vi "ATM Controller.vi"(8 "error in (no error)":errorcluster) -> (0 "error out":errorcluster)   [LabVIEW 2012]
uses:
  TypeDefs/ATM Controller State.ctl
  TypeDefs/UI Items.ctl
  TypeDefs/User Console Commands.ctl
  TypeDefs/Error Classification.ctl
  TypeDefs/Simulated Database Command.ctl
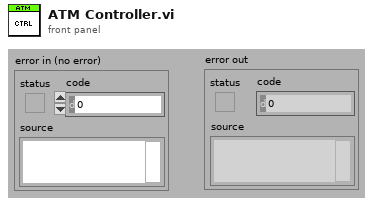
[diagram p1: front panel]
types:
  T1 = typedef "ATM Controller State.ctl" = enum16{"Initial", "Login", "Main Menu", "Balance Inquiry", "Deposit", "Deposit Complete", "Withdrawal", "Withdrawal Success", "Withdrawal Failure", "Terminate", "Lock Out"}
  T2 = typedef "User Console Commands.ctl" = enum16{"Init", "Set ATM Message", "Set ATM Menus", "Disable Controls", "Wait for Input", "Clear Keypad", "Return Card", "Close"}
  T3 = typedef "Error Classification.ctl" = enum16{"Minor", "Session", "System"}
  T4 = typedef "UI Items.ctl" = cluster{"Keypad":bool, "Card Slot":bool, "Left Buttons":bool, "Right Buttons":bool, "ATM Message":bool, "Left Menu":bool, "Right Menu":bool}
  T5 = typedef "Simulated Database Command.ctl" = enum16{"Init", "Look up and Lock Account", "Modify Balance", "Get Record", "Commit Record", "Unlock Record", "Close"}
  T6 = typedef "Record.ctl" = cluster{"Account Number":u32, "First Name":string, "Last Name":string, "Balance":dbl, "Locked":bool}
  T7 = typedef "UI to CTRL Command.ctl" = enum16{"Card Inserted", "Keypad Entry", "Button Pressed"}
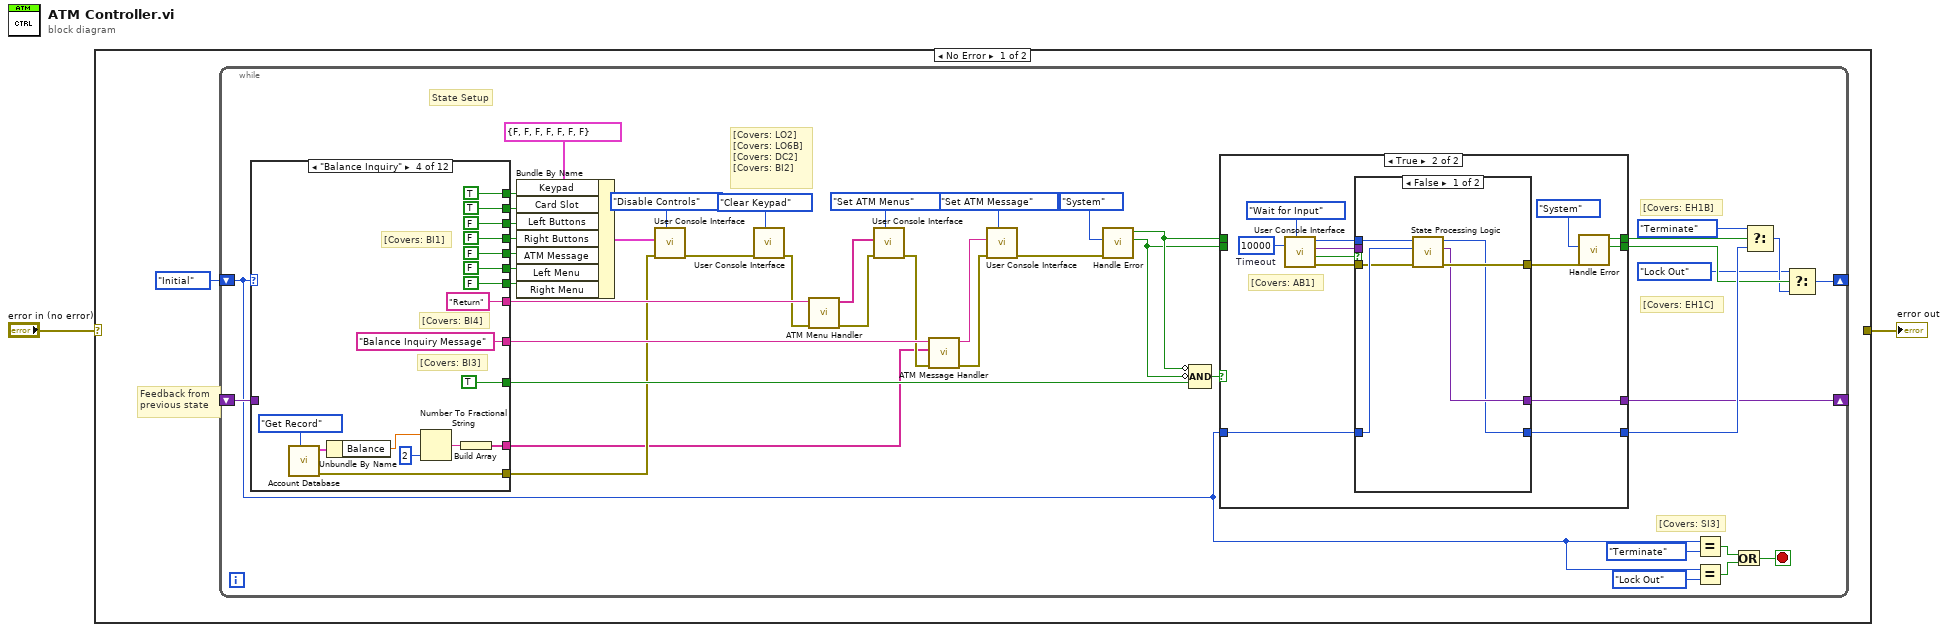
[diagram p0: block diagram]
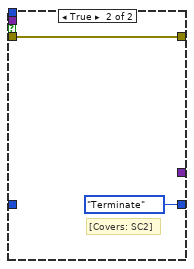
[diagram p3: hidden frame]
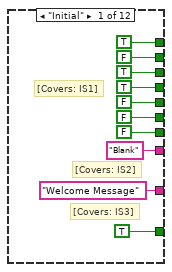
[diagram p4: hidden frame]
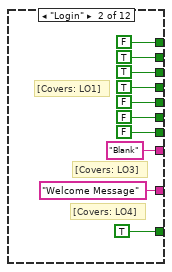
[diagram p5: hidden frame]
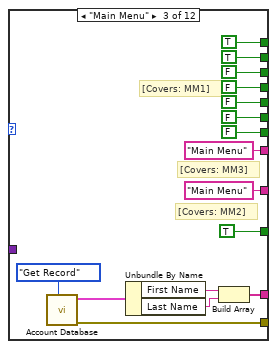
[diagram p6: hidden frame]
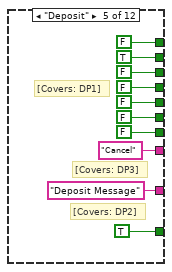
[diagram p7: hidden frame]
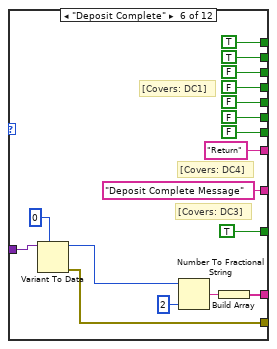
[diagram p8: hidden frame]
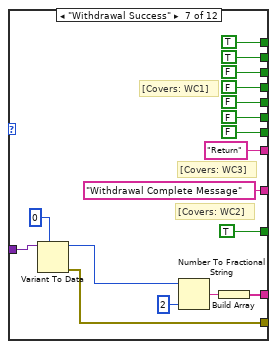
[diagram p9: hidden frame]
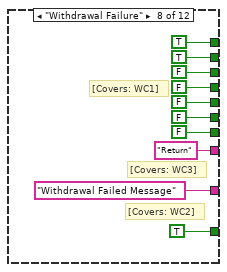
[diagram p10: hidden frame]
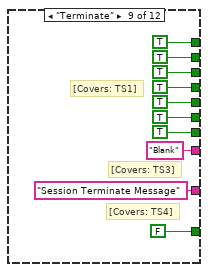
[diagram p11: hidden frame]
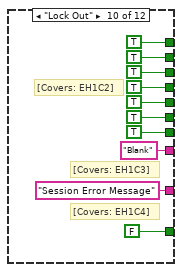
[diagram p12: hidden frame]
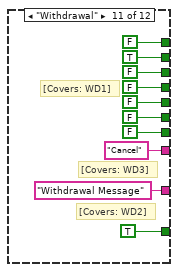
[diagram p13: hidden frame]
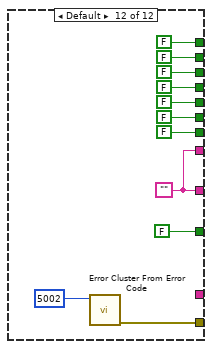
[diagram p14: hidden frame]
diagram:
  n1 = case shown="No Error" "error in (no error)" {
    selector: "error in (no error)" -> [_ w221]
    tunnel: [_ w221] -> w1
    frame No Error {
      # "Feedback from\nprevious state"
      n2 = while {
        shift-right: [w24] -> _
        shift-left: ATM_Controller_State."Initial" ("State") -> [w4]
        shift-right: [w11] -> _
        shift-left: _ -> [w10]
        stop <- w5 stop-if-true
        # "[Covers: SI3]"
        # "[Covers: LO2]\n[Covers: LO6B]\n[Covers: DC2]\n[Covers: BI2]"
        # "[Covers: EH1C]"
        # "[Covers: EH1B]"
        # "State Setup"
        n3 = case shown="\"Balance Inquiry\"" w4 {
          tunnel: [TRUE ("Keypad") FALSE ("Keypad") TRUE ("Keypad") TRUE ("Keypad") FALSE ("Keypad") TRUE ("Keypad") TRUE ("Keypad") TRUE ("Keypad") TRUE ("Keypad") TRUE ("Keypad") FALSE ("Keypad") FALSE ("Keypad")] -> w47
          tunnel: [FALSE ("Keypad") TRUE ("Keypad") TRUE ("Keypad") TRUE ("Keypad") TRUE ("Keypad") TRUE ("Keypad") TRUE ("Keypad") TRUE ("Keypad") TRUE ("Keypad") TRUE ("Keypad") TRUE ("Keypad") FALSE ("Keypad")] -> w46
          tunnel: [TRUE ("Keypad") TRUE ("Keypad") FALSE ("Keypad") FALSE ("Keypad") FALSE ("Keypad") FALSE ("Keypad") FALSE ("Keypad") FALSE ("Keypad") TRUE ("Keypad") TRUE ("Keypad") FALSE ("Keypad") FALSE ("Keypad")] -> w45
          tunnel: [TRUE ("Keypad") TRUE ("Keypad") FALSE ("Keypad") FALSE ("Keypad") FALSE ("Keypad") FALSE ("Keypad") FALSE ("Keypad") FALSE ("Keypad") TRUE ("Keypad") TRUE ("Keypad") FALSE ("Keypad") FALSE ("Keypad")] -> w44
          tunnel: [FALSE ("Keypad") FALSE ("Keypad") FALSE ("Keypad") FALSE ("Keypad") FALSE ("Keypad") FALSE ("Keypad") FALSE ("Keypad") FALSE ("Keypad") TRUE ("Keypad") TRUE ("Keypad") FALSE ("Keypad") FALSE ("Keypad")] -> w43
          tunnel: [FALSE ("Keypad") FALSE ("Keypad") FALSE ("Keypad") FALSE ("Keypad") FALSE ("Keypad") FALSE ("Keypad") FALSE ("Keypad") FALSE ("Keypad") TRUE ("Keypad") TRUE ("Keypad") FALSE ("Keypad") FALSE ("Keypad")] -> w42
          tunnel: [FALSE ("Keypad") FALSE ("Keypad") FALSE ("Keypad") FALSE ("Keypad") FALSE ("Keypad") FALSE ("Keypad") FALSE ("Keypad") FALSE ("Keypad") TRUE ("Keypad") TRUE ("Keypad") FALSE ("Keypad") FALSE ("Keypad")] -> w41
          tunnel: ["Blank" "Blank" "Main Menu" "Return" "Cancel" "Return" "Return" "Return" "Blank" "Blank" "Cancel" w212] -> w35
          tunnel: ["Welcome Message" "Welcome Message" "Main Menu" "Balance Inquiry Message" "Deposit Message" "Deposit Complete Message" "Withdrawal Complete Message" "Withdrawal Failed Message" "Session Terminate Message" "Session Error Message" "Withdrawal Message" w212] -> w38
          tunnel: [TRUE TRUE TRUE TRUE TRUE TRUE TRUE TRUE FALSE FALSE TRUE FALSE] -> w31
          tunnel: [_ _ w97 w114 _ w138 w155 _ _ _ _ w210] -> w13
          tunnel: [_ _ w93 w112 _ w142 w159 _ _ _ _ _] -> w12
          tunnel: w10 -> [_ _ _ _ _ w139 w156 _ _ _ _ _]
          frame "Initial" {
            # "[Covers: IS3]"
            # "[Covers: IS2]"
            # "[Covers: IS1]"
          }
          frame "Login" {
            # "[Covers: LO4]"
            # "[Covers: LO3]"
            # "[Covers: LO1]"
          }
          frame "Main Menu" {
            # "[Covers: MM2]"
            # "[Covers: MM3]"
            # "[Covers: MM1]"
            n4 = call "Account Database.vi"("Command"=Simulated_Database_Command."Get Record") -> ("error out"=w97:errorcluster, "Record"=w96:T6)  [unwired: 8 in, 1 out]
            n5 = Unbundle By Name(w96) -> ("First Name"=w95:string, "Last Name"=w94:string)
            n6 = Build Array(w95, w94) -> (w93:string[])
          }
          frame "Balance Inquiry" {
            # "[Covers: BI3]"
            # "[Covers: BI4]"
            # "[Covers: BI1]"
            n7 = call "Account Database.vi"("Command"=Simulated_Database_Command."Get Record") -> ("error out"=w114:errorcluster, "Record"=w113:T6)  [unwired: 8 in, 1 out]
            n8 = Unbundle By Name(w113) -> ("Balance"=w110:dbl)
            n9 = Number To Fractional String(number=w110, precision (6)=i16 2) -> (F-format string=w111:string)  [unwired: 2 in]
            n10 = Build Array(w111) -> (w112:string[])
          }
          frame "Deposit" {
            # "[Covers: DP2]"
            # "[Covers: DP3]"
            # "[Covers: DP1]"
          }
          frame "Deposit Complete" {
            # "[Covers: DC3]"
            # "[Covers: DC4]"
            # "[Covers: DC1]"
            n11 = Variant To Data(type=0, Variant=w139) -> (data=w136:i32, error out=w138:errorcluster)  [unwired: 1 in]
            n12 = Number To Fractional String(number=w136, precision (6)=i16 2) -> (F-format string=w141:string)  [unwired: 2 in]
            n13 = Build Array(w141) -> (w142:string[])
          }
          frame "Withdrawal Success" {
            # "[Covers: WC2]"
            # "[Covers: WC3]"
            # "[Covers: WC1]"
            n14 = Variant To Data(type=0, Variant=w156) -> (data=w153:i32, error out=w155:errorcluster)  [unwired: 1 in]
            n15 = Number To Fractional String(number=w153, precision (6)=i16 2) -> (F-format string=w158:string)  [unwired: 2 in]
            n16 = Build Array(w158) -> (w159:string[])
          }
          frame "Withdrawal Failure" {
            # "[Covers: WC2]"
            # "[Covers: WC3]"
            # "[Covers: WC1]"
          }
          frame "Terminate" {
            # "[Covers: TS4]"
            # "[Covers: TS3]"
            # "[Covers: TS1]"
          }
          frame "Lock Out" {
            # "[Covers: EH1C4]"
            # "[Covers: EH1C3]"
            # "[Covers: EH1C2]"
          }
          frame "Withdrawal" {
            # "[Covers: WD2]"
            # "[Covers: WD3]"
            # "[Covers: WD1]"
          }
          frame Default {
            w212 = "" ("Empty String Constant")
            n17 = call <vilib>:"Error Cluster From Error Code.vi"("error code (0)"=5002) -> ("error out"=w210:errorcluster)  [unwired: 8 in]
          }
        }
        n18 = Bundle By Name(cluster=T4 {"Keypad"=FALSE, "Card Slot"=FALSE, "Left Buttons"=FALSE, "Right Buttons"=FALSE, "ATM Message"=FALSE, "Left Menu"=FALSE, "Right Menu"=FALSE} ("UI Items"), "Keypad"=w47, "Card Slot"=w46, "Left Buttons"=w45, "Right Buttons"=w44, "ATM Message"=w43, "Left Menu"=w42, "Right Menu"=w41) -> (w19:T4)
        n19 = call "User Console Interface.vi"("Command"=User_Console_Commands."Disable Controls", "error in (no error)"=w13, "Parameter"=w19) -> ("error out"=w15:errorcluster)  [unwired: 5 in, 3 out]
        n20 = call "User Console Interface.vi"("Command"=User_Console_Commands."Clear Keypad", "error in (no error)"=w15) -> ("error out"=w14:errorcluster)  [unwired: 6 in, 3 out]
        n21 = call "ATM Menu Handler.vi"("error in (no error)"=w14, "Menu State"=w35) -> ("error out"=w34:errorcluster, "Menu Items"=w20:string[])  [unwired: 8 in]
        n22 = call "User Console Interface.vi"("Command"=User_Console_Commands."Set ATM Menus", "error in (no error)"=w34, "Parameter"=w20) -> ("error out"=w37:errorcluster)  [unwired: 5 in, 3 out]
        n23 = call "ATM Message Handler.vi"("error in (no error)"=w37, "Parameters"=w12, "Message Name"=w38) -> ("error out"=w36:errorcluster, "Message"=w21:string)  [unwired: 7 in]
        n24 = call "User Console Interface.vi"("Command"=User_Console_Commands."Set ATM Message", "error in (no error)"=w36, "Parameter"=w21) -> ("error out"=w33:errorcluster)  [unwired: 5 in, 3 out]
        n25 = call "Handle Error.vi"("error in (no error)"=w33, "Classification"=Error_Classification."System") -> ("System Error"=w29:bool, "Session Error"=w30:bool)  [unwired: 7 in, 1 out]
        n26 = Compound Arithmetic op=AND(invert w30, invert w29, w31) -> (w32:bool)
        n27 = case shown="True" w32 {
          tunnel: w30 -> [w51 _]
          tunnel: [w51 w56] -> w28
          tunnel: w29 -> [w50 _]
          tunnel: [w50 w55] -> w26
          tunnel: w4 -> [w49 w53]
          tunnel: [w49 w58] -> w27
          tunnel: [_ w52] -> w11
          frame False {
          }
          frame True {
            w63 = 10000  # Timeout
            # "[Covers: AB1]"
            n28 = call "User Console Interface.vi"("Command"=User_Console_Commands."Wait for Input", "Parameter"=w63) -> ("error out"=w60:errorcluster, "timed out?"=w62:bool, "Parameter Out"=w59:variant, "User Input"=w61:T7)  [unwired: 6 in]
            n29 = case shown="False" w62 {
              tunnel: w61 -> [w69 _]
              tunnel: w60 -> [w68 w71]
              tunnel: w59 -> [_ _]
              tunnel: [w65 ATM_Controller_State."Terminate" ("State")] -> w58
              tunnel: [w67 w71] -> w54
              tunnel: w53 -> [w70 _]
              tunnel: [w66 _] -> w52
              frame False {
                n30 = call "State Processing Logic.vi"("error in"=w68, "Parameter"=w70, "User Input"=w69) -> ("error out"=w67:errorcluster, "Feedback"=w66:variant, "State Out"=w65:T1)  [unwired: 6 in]
              }
              frame True {
                # "[Covers: SC2]"
              }
            }
            n31 = call "Handle Error.vi"("error in (no error)"=w54, "Classification"=Error_Classification."System") -> ("System Error"=w55:bool, "Session Error"=w56:bool)  [unwired: 7 in, 1 out]
          }
        }
        n32 = Equal?(x=w4, y=ATM_Controller_State."Terminate") -> (x = y?=w6:bool)
        n33 = Equal?(x=w4, y=ATM_Controller_State."Lock Out") -> (x = y?=w7:bool)
        n34 = Or(x=w6, y=w7) -> (x .or. y?=w5:bool)
        n35 = Select(t=ATM_Controller_State."Terminate", s=w28, f=w27) -> (s? t:f=w25:T1)
        n36 = Select(t=ATM_Controller_State."Lock Out", s=w26, f=w25) -> (s? t:f=w24:T1)
      }
    }
    frame Error {
    }
  }
  "error out" <- w1
